vi "GoldenBackground kopieren.vi"(11 "error in (no error)":errorcluster caption="Fehler (Eingang, kein Fehler)") -> (15 "error out":errorcluster caption="Fehler (Ausgang)")   [LabVIEW 2020, in "FT-IR.lvlib" / "Get Spectra.lvlib"]
uses:
  Get Spectra.lvlib
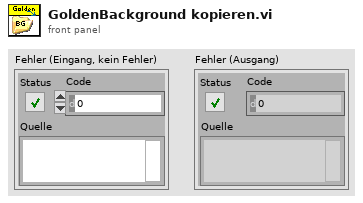
[diagram p1: front panel]
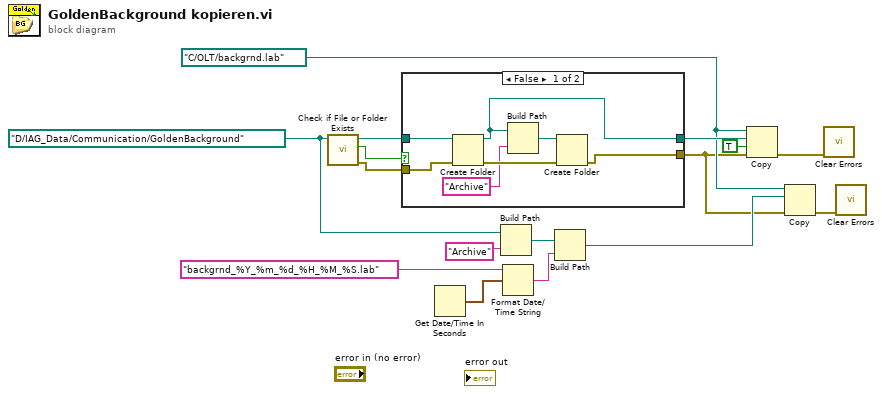
[diagram p0: block diagram]
diagram:
  w5 = path "C:/OLT/backgrnd.lab" ("Quellpfad")
  w9 = path "D:/IAG_Data/Communication/GoldenBackground" ("path")
  n1 = call <vilib>:"Check if File or Folder Exists.vi"("path"=w9) -> ("error out"=w11:errorcluster, "file or folder exists?"=w13:bool, "dup path"=w14:path)  [unwired: 8 in]
  n2 = case shown="False" w13 {
    tunnel: w14 -> [w23 w25]
    tunnel: [w17 w25] -> w12
    tunnel: w11 -> [w22 w24]
    tunnel: [w18 w24] -> w3
    frame False {
      n3 = Create Folder(path (use dialog)=w23, error in=w22) -> (created path=w17:path, error out=w21:errorcluster)  [unwired: 1 in, 1 out]
      n4 = Build Path(base path=w17, name or relative path="Archive") -> (appended path=w20:path)
      n5 = Create Folder(path (use dialog)=w20, error in=w21) -> (error out=w18:errorcluster)  [unwired: 1 in, 2 out]
    }
    frame True {
    }
  }
  n6 = Get Date/Time In Seconds() -> (seconds since 1Jan1904=w16:timestamp)
  n7 = Build Path(base path=w9, name or relative path="Archive") -> (appended path=w7:path)
  n8 = Format Date/Time String(time format string (%c)="backgrnd_%Y_%m_%d_%H_%M_%S.lab" ("Zeitformatierungs-String (%c)"), seconds (now)=w16) -> (date/time string=w6:string)  [unwired: 1 in]
  n9 = Build Path(base path=w7, name or relative path=w6) -> (appended path=w4:path)
  n10 = Copy(8:w3, 9:TRUE ("Überschreiben (F)"), 10:w12, 11:w5) -> (0:w10:errorcluster)  [unwired: 1 in, 2 out]
  n11 = Copy(8:w3, 10:w4, 11:w5) -> (0:w2:errorcluster)  [unwired: 2 in, 2 out]
  n12 = call <vilib>:"Clear Errors.vi"("error in (no error)"=w10) -> ()  [unwired: 5 in, 2 out]
  n13 = call <vilib>:"Clear Errors.vi"("error in (no error)"=w2) -> ()  [unwired: 5 in, 2 out]
